vi "test.vi"   [LabVIEW 2017]
uses:
  4d204507-ace2-4824-bd05-8510f7e641a2.vi
  src/TagDB/_Support/DataAccess/data-Write.vi
  src/TagDB/_Support/Error/_[error50000]Invalid DB REF.vi
  src/TagDB/_Support/DataAccess/TagDB Ref to DVR.vi
  src/TagDB/_Support/DataAccess/_NameCacher.vi
  src/TagDB/_Support/DataAccess/_datatypeChecker.vi
  <vilib>/Utility/Data Type/Get Type Information.vi
  src/TagDB/_Support/Error/_Build Error Cluster.vi
  src/TagDB/TagDB.lvlib
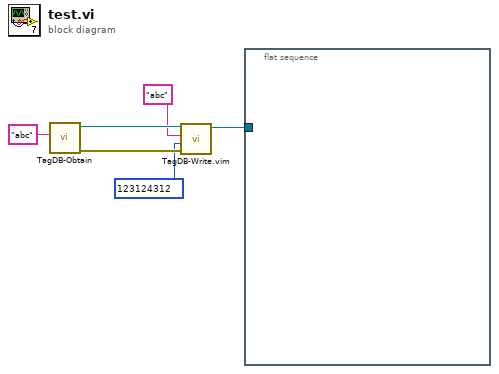
[diagram p0: block diagram]
diagram:
  n1 = call "TagDB-Obtain.vi"("name (unnamed)"="abc") -> ("error out"=w4:errorcluster, "TagDB"=w5:refnum<k1>)  [unwired: 4 in, 1 out]
  n2 = call "TagDB-Write.vim"("error in (no error)"=w4, "Value"=123124312, "tag"="abc", "TagDB"=w5) -> ("TagDB(dup)"=w1:refnum<k1>)  [unwired: 5 in, 2 out]
  n3 = flat-sequence {
    tunnel: w1 -> [_]
    frame #0 {
    }
  }
